vi "TPDO RPDO.vi"() -> (1 "TPDO":T1[](array[typedef]) format="%.0x", 2 "RPDO":dbl[](array[numeric]) format="%.2f")   [LabVIEW 2013]
uses:
  <vilib>/NI Veristand/Custom Device API/Data Reference.ctl
  Global debug.vi
  <vilib>/NI Veristand/Custom Device API/Custom Device API.lvlib
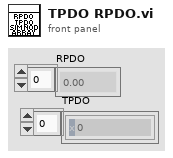
[diagram p1: front panel]
types:
  T1 = typedef "Custom Device API.lvlib/Data Reference.ctl" = i32
  T2 = typedef "CANOpen_Settings.ctl" = cluster{"Driver Settings":T3, "Data References":T17, "Bus Commands":T19, "SDO Asynch":T20, "Status NMT":T21}
  T3 = typedef "CANOpen_Node Settings.ctl" = cluster{"CANOpen Bus Settings":T4, "Nodes":T7[], "Node Ids":T16}
  T4 = typedef "CANOpen Addon Custom Device.lvlib/CANOpen_Bus Settings.ctl" = cluster{"CANOpen Interface Name":T5, "Baud Rate":T6, "Termination":bool, "Sync Period (ms)":i64, "Enable 9881":bool, "RIO Device":u16, "Enable SYNC":bool, "Scan & Print":bool}
  T5 = typedef "CANOpen Addon Custom Device.lvlib/CANOpen Interface Name.ctl" = u32
  T6 = typedef "CANopen BaudRate.ctl" = u32
  T7 = typedef "CANOpen_Node Message Settings.ctl" = cluster{"RPDOs":T8[], "TPDOs":T8[], "Node ID":u8, "SDOs":T12[], "Dynamic SDOs":T12[], "NMT":T13}
  T8 = typedef "CANOpen Addon Custom Device.lvlib/CANOpen_PDO Settings.ctl" = cluster{"Parameters":T9[], "PDO Channel":u8, "Start Index":u32, "Length":u32}
  T9 = typedef "CANOpen Addon Custom Device.lvlib/CANOpen_PDO Parameter Settings.ctl" = cluster{"Parameter Name":string, "Scale Factor":dbl, "Scale Offset":dbl, "Byte Offset":u8, "Bit Offset":u8, "Data Type":T10, "Byte Order":T11}
  T10 = typedef "CANOpen Addon Custom Device.lvlib/CANOpen_PDO Data Type.ctl" = enum16{"U8", "U16", "U32", "I8", "I16", "I32", "Single", "Double", "Boolean"}
  T11 = typedef "CANOpen Addon Custom Device.lvlib/CANopen Byte Order.ctl" = enum16{"big-endian network order", "little-endian"}
  T12 = typedef "CANOpen Addon Custom Device.lvlib/CANOpen_SDO Settings.ctl" = cluster{"Object Index":u16, "Sub-Index (0)":u8, "Block Data":u8[], "Name":string}
  T13 = typedef "CANOpen Addon Custom Device.lvlib/CANOpen_NMT Settings.ctl" = cluster{"Node run state":u16, "Emergency":bool, "HB NG":T14, "Delay for opp. state (ms)":dbl, "Node init static SDO state":u16, "Stop and Reset on Shutdown":bool}
  T14 = typedef "CANOpen Addon Custom Device.lvlib/CanOpen_NMT_Config.ctl" = cluster{"Mode":T15, "Update Time":u16, "Static detect in None":T15}
  T15 = typedef "CANOpen Addon Custom Device.lvlib/CanOpen_NMT_Static detect.ctl" = enum16{"None", "HB", "NG"}
  T16 = typedef "CANOpen Addon Custom Device.lvlib/CanOpen_Main Node Ids.ctl" = u8[]
  T17 = typedef "CANOpen_VS Data Refs.ctl" = cluster{"Hardware Input":cluster{"FIFO":refnum<k33>, "Channel Pairs":cluster{"Chan Refs":T1[], "Prev. Values":dbl[]}}, "Hardware Output":cluster{"FIFO":refnum<k33>, "Channel Pairs":cluster{"Block Refs":T18[], "Prev. Values":dbl[]}}}
  T18 = typedef "Custom Device API.lvlib/Block Data Reference.ctl" = cluster{"Data Reference":T1, "Offset":i32, "Length":i32}
  T19 = typedef "CANOpen_VS Bidirectional Data Refs.ctl" = cluster{"Hardware Output":cluster{"FIFO":refnum<k33>, "Channel Pairs":cluster{"Chan Refs":T1[], "Prev. Values":dbl[]}}, "Hardware Input":cluster{"FIFO":refnum<k33>}}
  T20 = typedef "CANOpen Addon Custom Device.lvlib/CANOpen_VS SDOs Data Refs.ctl" = cluster{"List SDO":cluster{"FIFO Req":refnum<k33>, "Req Chan.":cluster{"Chan Refs":T1[], "NodeIndex":dbl[]}, "FIFO Resp":refnum<k33>, "Resp Chan.":cluster{"Chan Refs":T1[]}, "Node IDs":u8[], "FIFO array":dbl[]}, "HW Dyn Write":cluster{"FIFO Req":refnum<k33>, "FIFO Resp":refnum<k33>, "Req Chan.":cluster{"Chan Refs":T1[], "Node IDs":u8[]}, "Resp Chan.":cluster{"Chan Refs":T1[]}}, "HW Dyn Read":cluster{"FIFO Req":refnum<k33>, "FIFO Resp":refnum<k33>, "Req Chan.":cluster{"Chan Refs":T1[], "Node IDs":u8[]}, "Resp Chan.":cluster{"Chan Refs":T1[]}}}
  T21 = typedef "CANOpen Addon Custom Device.lvlib/CANOpen_VS Status Management Data Refs.ctl" = cluster{"Hardware Output":cluster{"FIFO":refnum<k33>, "Channel Pairs":T22}, "Hardware Input":cluster{"FIFO":refnum<k33>, "Channel Pairs":T23}}
  T22 = typedef "CANOpen Addon Custom Device.lvlib/CanOpen_NMT_HWOut_ChannelPairs.ctl" = cluster{"Chan Refs":T18[], "Prev. Values":dbl[], "Node index":dbl[]}
  T23 = typedef "CANOpen Addon Custom Device.lvlib/CanOpen_NMT_HWIn_ChannelPairs.ctl" = cluster{"Chan Refs":T1[], "Prev. Values":dbl[], "Node index":dbl[]}
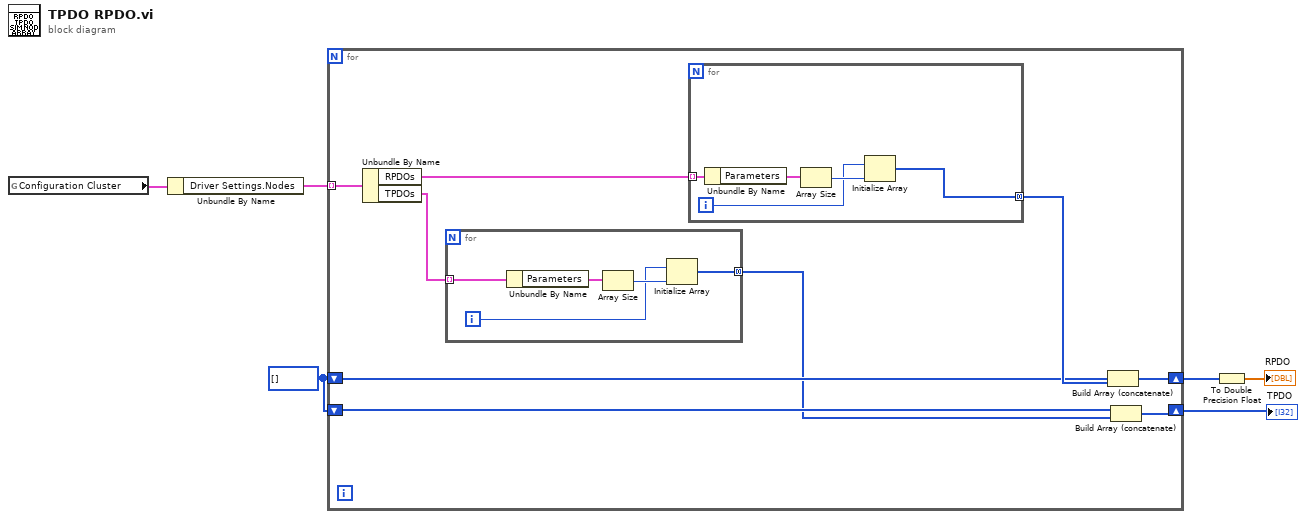
[diagram p0: block diagram]
diagram:
  w4 = T1[] []
  n1 = global read "Global debug.vi" "Configuration Cluster"() -> (w6:T2)
  n2 = Unbundle By Name(w6) -> ("Driver Settings.Nodes"=w5:T7[])
  n3 = for {
    tunnel: w5 -> [w15] mode=indexing
    shift-right: [w8] -> w3
    shift-left: w4 -> [w12]
    shift-right: [w7] -> w1
    shift-left: w4 -> [w10]
    n4 = Unbundle By Name(w15) -> ("RPDOs"=w14:T8[], "TPDOs"=w11:T8[])
    n5 = for {
      tunnel: w11 -> [w18] mode=indexing
      tunnel: [w16] -> w9 mode=concatenating
      i -> [w17]
      n6 = Unbundle By Name(w18) -> ("Parameters"=w19:T9[])
      n7 = Array Size(array=w19) -> (size(s)=w20:i32)
      n8 = Initialize Array(w17, w20) -> (w16:i32[])
    }
    n9 = for {
      tunnel: w14 -> [w25] mode=indexing
      tunnel: [w21] -> w13 mode=concatenating
      i -> [w22]
      n10 = Unbundle By Name(w25) -> ("Parameters"=w24:T9[])
      n11 = Array Size(array=w24) -> (size(s)=w23:i32)
      n12 = Initialize Array(w22, w23) -> (w21:i32[])
    }
    n13 = Build Array (concatenate)(w12, w13) -> (w8:T1[])
    n14 = Build Array (concatenate)(w10, w9) -> (w7:T1[])
  }
  "TPDO" <- w1
  n15 = To Double Precision Float(number=w3) -> (double precision float=→"RPDO":dbl[])
